vi "myRIO_BRig_RT_dataMTrig_Laser_c.vi"() -> (2 "output_Laser_c":i32)   [LabVIEW 2014]
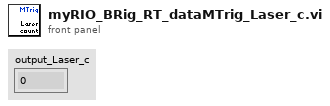
[diagram p1: front panel]
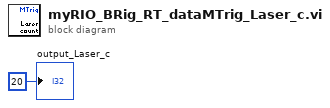
[diagram p0: block diagram]
diagram:
  "output_Laser_c" <- 20 ("output_iBlock")
